vi "Read Index.vi"(8 "error in (no error)":errorcluster, 11 "Card in":refnum<class "Card.lvclass">) -> (0 "error out":errorcluster, 2 "Index":i32, 3 "Card out":refnum<class "Card.lvclass">)   [LabVIEW 2020, in "Card.lvclass"]
uses:
  Card.lvclass
  Card.lvclass/Card.ctl
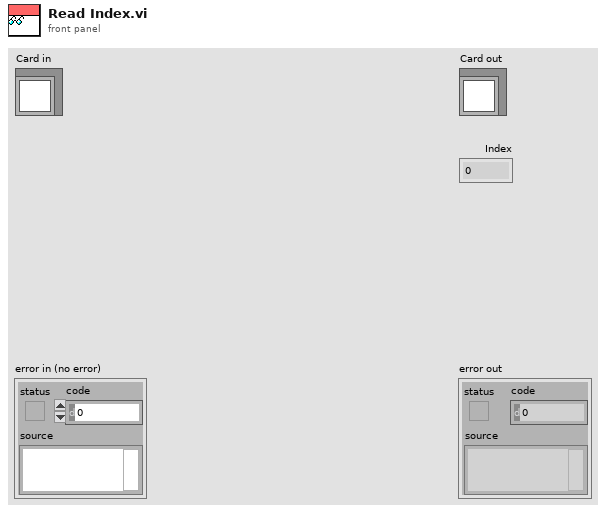
[diagram p1: front panel]
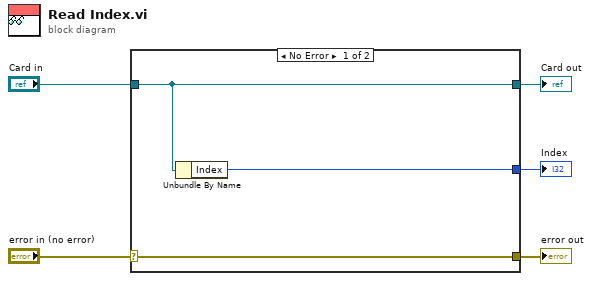
[diagram p0: block diagram]
diagram:
  n1 = case shown="No Error" "error in (no error)" {
    selector: "error in (no error)" -> [w8 w9]
    tunnel: [w8 w9] -> w4
    tunnel: [w7 w10] -> w2
    tunnel: "Card in" -> [w7 w10]
    tunnel: [w6 _] -> w1
    frame No Error {
      n2 = Unbundle By Name(w7) -> ("Index"=w6:i32)
    }
    frame Error {
    }
  }
  "error out" <- w4
  "Card out" <- w2
  "Index" <- w1
